vi "UniquifyFullyQualifiedVIName.vi"(8 "error in (no error)":errorcluster, 10 "suffix":string="_COPY", 11 "vi path":path) -> (0 "error out":errorcluster, 3 "uniquified vi path":path)   [LabVIEW 2015, in "UniquifyFullyQualifiedVIName.lvclass"]
uses:
  UniquifyFullyQualifiedVIName.lvclass
  <vilib>/regexp/Match Regular Expression.xnode
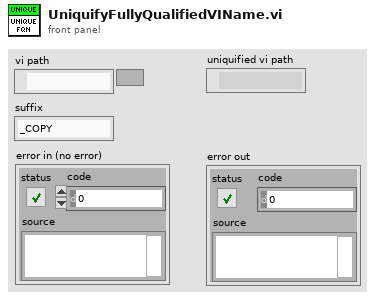
[diagram p1: front panel]
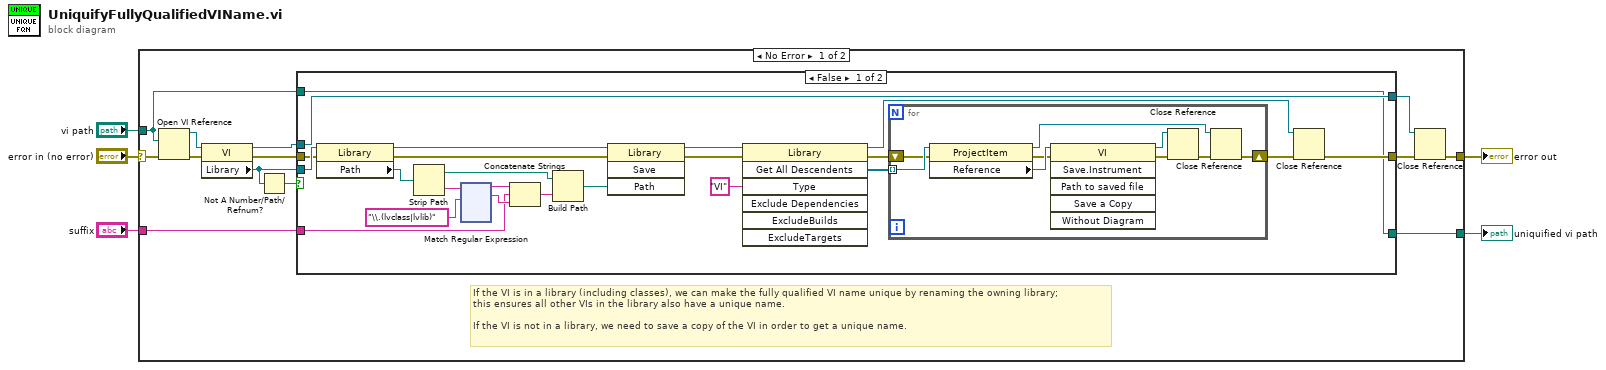
[diagram p0: block diagram]
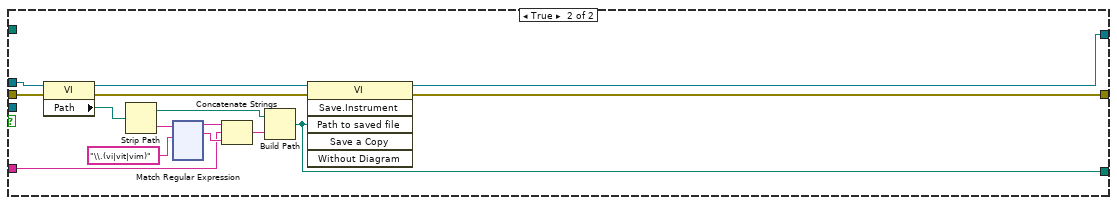
[diagram p2: hidden frame]
diagram:
  n1 = case shown="No Error" "error in (no error)" {
    selector: "error in (no error)" -> [w15 w294]
    tunnel: "vi path" -> [w6 _]
    tunnel: [w13 w294] -> w3
    tunnel: "suffix" -> [w12 _]
    tunnel: [w7 _] -> w1
    frame No Error {
      # "If the VI is in a library (including classes), we can make the fully qualified VI name unique by renaming the owning library;\nthis ensures all other VIs in the library also have a unique name.\n\nIf the VI is not in a library, we need to save a copy of the VI in order to get a unique name."
      n2 = Open VI Reference(vi path=w6, error in (no error)=w15) -> (vi reference=w18:refnum<vi>, error out=w16:errorcluster)  [unwired: 4 in]
      n3 = property class="VI"(reference=w18, error in=w16) -> (reference out=w9:refnum<vi>, error out=w17:errorcluster, "Library"=w11:refnum<vi>)
      n4 = Not A Number/Path/Refnum?(number/path/refnum=w11) -> (NaN/Path/Refnum?=w10:bool)
      n5 = case shown="False" w10 {
        tunnel: w11 -> [w37 _]
        tunnel: w17 -> [w30 w170]
        tunnel: [w22 w166] -> w14
        tunnel: w12 -> [w21 w168]
        tunnel: w9 -> [w20 w172]
        tunnel: [w20 w179] -> w8
        tunnel: [w19 w165] -> w7
        tunnel: w6 -> [w19 _]
        frame False {
          n6 = property class="Library"(reference=w37, error in=w30) -> (reference out=w36:refnum<vi>, error out=w31:errorcluster, "Path"=w41:path)
          n7 = Strip Path(path=w41) -> (stripped path=w40:path, name=w28:string)
          n8 = xnode "Match Regular Expression"("input string"=w28, "regular expression"="\\.(lvclass|lvlib)") -> ("before match"=w27:string, "whole match"=w26:string)  [unwired: 4 in, 3 out]
          n9 = Concatenate Strings(w27, w21, w26) -> (w25:string)
          n10 = Build Path(base path=w40, name or relative path=w25) -> (appended path=w39:path)
          n11 = invoke class="Library" method="Save"(reference=w36, error in=w31, "Path"=w39) -> (reference out=w38:refnum<vi>, error out=w32:errorcluster)  [unwired: 1 in, 2 out]
          n12 = invoke class="Library" method="Get All Descendents"(reference=w38, error in=w32, "Type"="VI") -> (reference out=w23:refnum<vi>, error out=w33:errorcluster, "All Descendents"=w35:refnum<vi>[])  [unwired: 4 in, 4 out]
          n13 = for {
            tunnel: w35 -> [w163] mode=indexing
            shift-right: [w157] -> w24
            shift-left: w33 -> [w161]
            n14 = property class="ProjectItem"(reference=w163, error in=w161) -> (reference out=w156:refnum<vi>, error out=w162:errorcluster, "Reference"=w164:refnum<vi>)
            n15 = invoke class="VI" method="Save.Instrument"(reference=w164, error in=w162) -> (reference out=w159:refnum<vi>, error out=w160:errorcluster)  [unwired: 4 in, 4 out]
            n16 = Close Reference(reference=w159, error in (no error)=w160) -> (error out=w158:errorcluster)
            n17 = Close Reference(reference=w156, error in (no error)=w158) -> (error out=w157:errorcluster)
          }
          n18 = Close Reference(reference=w23, error in (no error)=w24) -> (error out=w22:errorcluster)
        }
        frame True {
          n19 = property class="VI"(reference=w172, error in=w170) -> (reference out=w171:refnum<vi>, error out=w167:errorcluster, "Path"=w169:path)
          n20 = Strip Path(path=w169) -> (stripped path=w178:path, name=w176:string)
          n21 = xnode "Match Regular Expression"("input string"=w176, "regular expression"="\\.(vi|vit|vim)") -> ("before match"=w175:string, "whole match"=w174:string)  [unwired: 4 in, 3 out]
          n22 = Concatenate Strings(w175, w168, w174) -> (w173:string)
          n23 = Build Path(base path=w178, name or relative path=w173) -> (appended path=w165:path)
          n24 = invoke class="VI" method="Save.Instrument"(reference=w171, error in=w167, "Path to saved file"=w165) -> (reference out=w179:refnum<vi>, error out=w166:errorcluster)  [unwired: 3 in, 4 out]
        }
      }
      n25 = Close Reference(reference=w8, error in (no error)=w14) -> (error out=w13:errorcluster)
    }
    frame Error {
    }
  }
  "error out" <- w3
  "uniquified vi path" <- w1
